vi "init.vi"(2 "error in (no error)":errorcluster) -> (0 "error out":errorcluster)   [LabVIEW 2016]
uses:
  <vilib>/SmarAct/MCS/Types/mcsSensorTypes.ctl
  sa commands.ctl
panel:
  out "Rotation channel":u32
  out "Y channel":u32=2
  out "X channel":u32=1
  out "System Index":u32=35
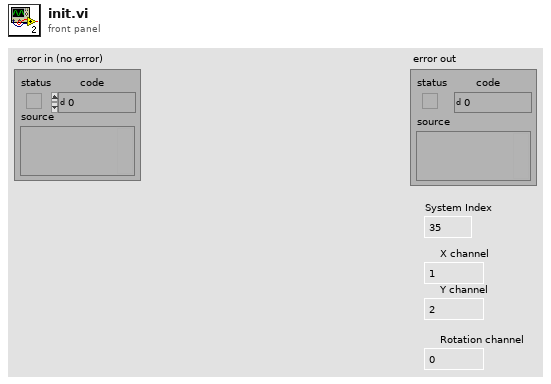
[diagram p1: front panel]
types:
  T1 = enum32{"SA_NO_REPORT_ON_COMPLETE", "SA_REPORT_ON_COMPLETE"}
  T2 = typedef "sa commands.ctl" = enum16{"read all", "set system index", "set x channel", "set y channel", "set rotation channel"}
  T3 = typedef "mcsSensorTypes.ctl" = enum32{"SA_NO_SENSOR_TYPE", "SA_S_SENSOR_TYPE", "SA_SR_SENSOR_TYPE", "SA_ML_SENSOR_TYPE", "SA_MR_SENSOR_TYPE", "SA_SP_SENSOR_TYPE", "SA_SC_SENSOR_TYPE", "SA_M25_SENSOR_TYPE", "SA_SR20_SENSOR_TYPE", "SA_M_SENSOR_TYPE", "SA_GC_SENSOR_TYPE", "SA_GD_SENSOR_TYPE", "SA_GE_SENSOR_TYPE", "SA_RA_SENSOR_TYPE", "SA_GF_SENSOR_TYPE", "SA_RB_SENSOR_TYPE", "SA_G605S_SENSOR_TYPE", "SA_G775S_SENSOR_TYPE", "SA_SC500_SENSOR_TYPE", "SA_G955S_SENSOR_TYPE", "SA_SR77_SENSOR_TYPE", "SA_SD_SENSOR_TYPE", "SA_R20ME_SENSOR_TYPE", "SA_SR2_SENSOR_TYPE", "SA_SCD_SENSOR_TYPE", "SA_SRC_SENSOR_TYPE", "SA_SR36M_SENSOR_TYPE", "SA_SR36ME_SENSOR_TYPE", "SA_SR50M_SENSOR_TYPE", "SA_SR50ME_SENSOR_TYPE", "SA_G1045S_SENSOR_TYPE", "SA_G1395S_SENSOR_TYPE", "SA_MD_SENSOR_TYPE", "SA_G935M_SENSOR_TYPE", "SA_SHL20_SENSOR_TYPE", "SA_SCT_SENSOR_TYPE", "SA_SR77T_SENSOR_TYPE", "SA_SR120_SENSOR_TYPE", "SA_LC_SENSOR_TYPE", "SA_LR_SENSOR_TYPE", "SA_LCD_SENSOR_TYPE", "SA_L_SENSOR_TYPE", "SA_LD_SENSOR_TYPE", "SA_LE_SENSOR_TYPE", "SA_LED_SENSOR_TYPE", "SA_GDD_SENSOR_TYPE", "SA_GED_SENSOR_TYPE", "SA_G935S_SENSOR_TYPE", "SA_G605DS_SENSOR_TYPE", "SA_G775DS_SENSOR_TYPE"}
  T4 = enum32{"SA_SENSOR_DISABLED", "SA_SENSOR_ENABLED", "SA_SENSOR_POWERSAVE"}
  T5 = enum32{"SA_UNBUFFERED_OUTPUT", "SA_BUFFERED_OUTPUT"}
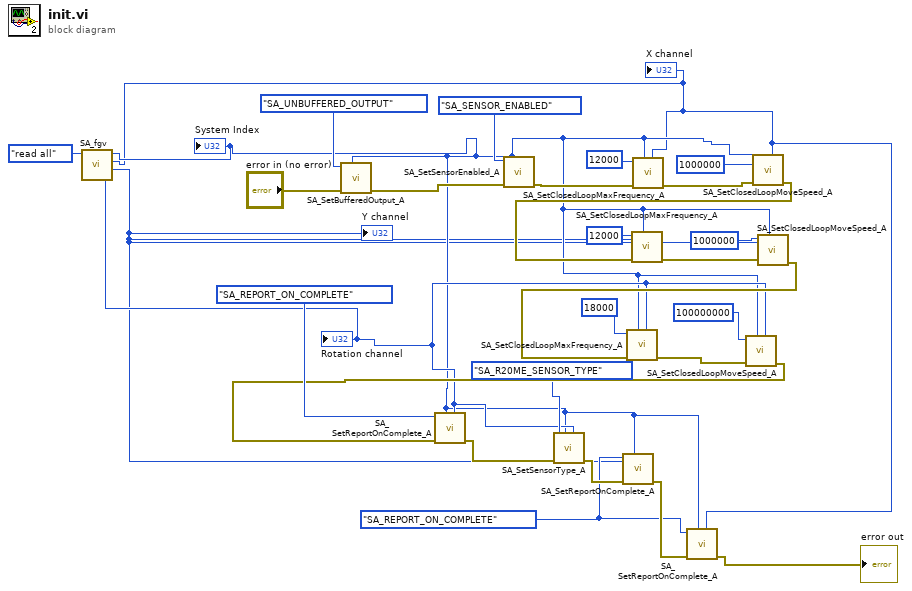
[diagram p0: block diagram]
diagram:
  w5 = T1."SA_REPORT_ON_COMPLETE" ("report")
  n1 = call "SA_fgv.vi"("command"=sa_commands."read all") -> ("rotation channel"=w9:u32, "y channel"=w3:u32, "x channel"=w2:u32, "system index"=w4:u32)  [unwired: 3 in]
  "System Index" <- w4
  "X channel" <- w2
  "Y channel" <- w3
  "Rotation channel" <- w9
  n2 = call <vilib>:"SA_SetBufferedOutput_A.vi"("systemIndex"=w4, "error in (no error)"="error in (no error)", "mode"=T5."SA_UNBUFFERED_OUTPUT") -> ("error out"=w16:errorcluster)  [unwired: 8 in]
  n3 = call <vilib>:"SA_SetSensorEnabled_A.vi"("systemIndex"=w4, "error in (no error)"=w16, "enabled"=T4."SA_SENSOR_ENABLED") -> ("error out"=w19:errorcluster)  [unwired: 8 in]
  n4 = call <vilib>:"SA_SetClosedLoopMaxFrequency_A.vi"("channelIndex"=w2, "systemIndex"=w4, "error in (no error)"=w19, "frequency"=u32 12000) -> ("error out"=w26:errorcluster)  [unwired: 7 in]
  n5 = call <vilib>:"SA_SetClosedLoopMoveSpeed_A.vi"("channelIndex"=w2, "systemIndex"=w4, "error in (no error)"=w26, "speed"=u32 1000000) -> ("error out"=w15:errorcluster)  [unwired: 7 in]
  n6 = call <vilib>:"SA_SetClosedLoopMaxFrequency_A.vi"("channelIndex"=w3, "systemIndex"=w4, "error in (no error)"=w15, "frequency"=u32 12000) -> ("error out"=w28:errorcluster)  [unwired: 7 in]
  n7 = call <vilib>:"SA_SetClosedLoopMoveSpeed_A.vi"("channelIndex"=w3, "systemIndex"=w4, "error in (no error)"=w28, "speed"=u32 1000000) -> ("error out"=w14:errorcluster)  [unwired: 7 in]
  n8 = call <vilib>:"SA_SetClosedLoopMaxFrequency_A.vi"("channelIndex"=w9, "systemIndex"=w4, "error in (no error)"=w14, "frequency"=u32 18000) -> ("error out"=w29:errorcluster)  [unwired: 7 in]
  n9 = call <vilib>:"SA_SetClosedLoopMoveSpeed_A.vi"("channelIndex"=w9, "systemIndex"=w4, "error in (no error)"=w29, "speed"=u32 100000000) -> ("error out"=w13:errorcluster)  [unwired: 7 in]
  n10 = call <vilib>:"SA_SetReportOnComplete_A.vi"("channelIndex"=w9, "systemIndex"=w4, "error in (no error)"=w13, "report"=T1."SA_REPORT_ON_COMPLETE") -> ("error out"=w11:errorcluster)  [unwired: 7 in]
  n11 = call <vilib>:"SA_SetSensorType_A.vi"("channelIndex"=w9, "systemIndex"=w4, "error in (no error)"=w11, "type"=mcsSensorTypes."SA_R20ME_SENSOR_TYPE") -> ("error out"=w7:errorcluster)  [unwired: 7 in]
  n12 = call <vilib>:"SA_SetReportOnComplete_A.vi"("channelIndex"=w3, "systemIndex"=w4, "error in (no error)"=w7, "report"=w5) -> ("error out"=w6:errorcluster)  [unwired: 7 in]
  n13 = call <vilib>:"SA_SetReportOnComplete_A.vi"("channelIndex"=w2, "systemIndex"=w4, "error in (no error)"=w6, "report"=w5) -> ("error out"=→"error out":errorcluster)  [unwired: 7 in]
